vi "niFpga wdp fft output fifo boolean.vi"(9 "enable":bool, 10 "enable with delay":bool, 11 "boolean in":bool) -> (3 "boolean out":bool)   [LabVIEW 2017]
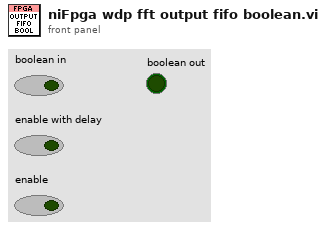
[diagram p1: front panel]
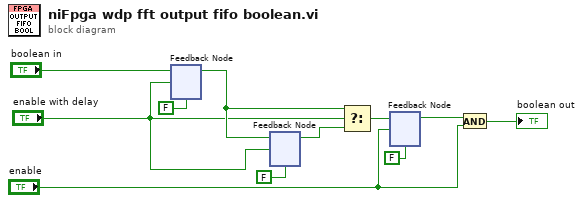
[diagram p0: block diagram]
diagram:
  n1 = feedback #1(FALSE ("boolean in")) -> (w9:bool)
  n2 = feedback-in #1("boolean in", "enable with delay") -> ()
  n3 = feedback #2(FALSE ("boolean in")) -> (w10:bool)
  n4 = feedback-in #2(w9, "enable with delay") -> ()
  n5 = Select(t=w9, s="enable with delay", f=w10) -> (s? t:f=w11:bool)
  n6 = feedback #3(FALSE ("boolean in")) -> (w3:bool)
  n7 = feedback-in #3(w11, "enable") -> ()
  n8 = And(x=w3, y="enable") -> (x .and. y?=→"boolean out":bool)
